vi "chart set up down bars format.vi"(0 "chart":u32, 1 "down_bar_fill":T1, 5 "up_bar_line":T2, 7 "up_bar_fill":T1, 9 "down_bar_line":T2, 11 "error in (no error)":errorcluster) -> (3 "down_bar_fill out":T1, 6 "up_bar_line out":T2, 8 "up_bar_fill out":T1, 10 "down_bar_line out":T2, 15 "error out":errorcluster)   [LabVIEW 2015, in "xlsxwriter.lvlib"]
doc: "void chart_set_up_down_bars_format(lxw_chart chart, lxw_chart_line *up_bar_line, lxw_chart_fill *up_bar_fill, lxw_chart_line *down_bar_line, lxw_chart_fill *down_bar_fill);"
uses:
  xlsxwriter.lvlib
  xlsxwriter.dll
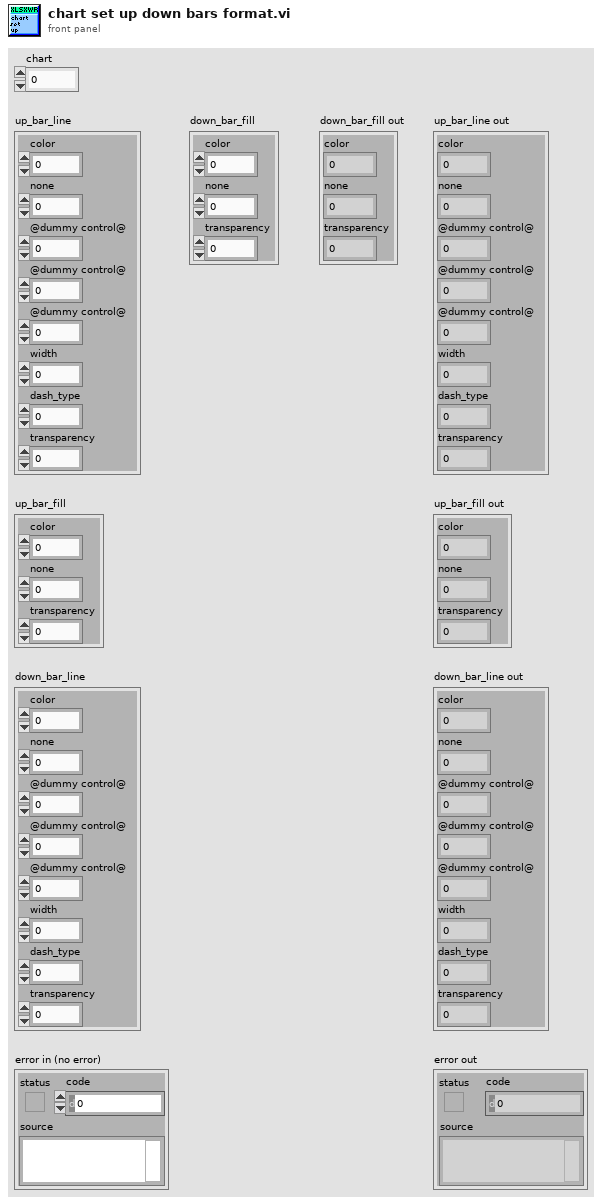
[diagram p1: front panel]
types:
  T1 = cluster{"color":u32, "none":u8, "transparency":u8}
  T2 = cluster{"color":u32, "none":u8, "@dummy control@":i8, "@dummy control@":i8, "@dummy control@":i8, "width":sgl, "dash_type":u8, "transparency":u8}
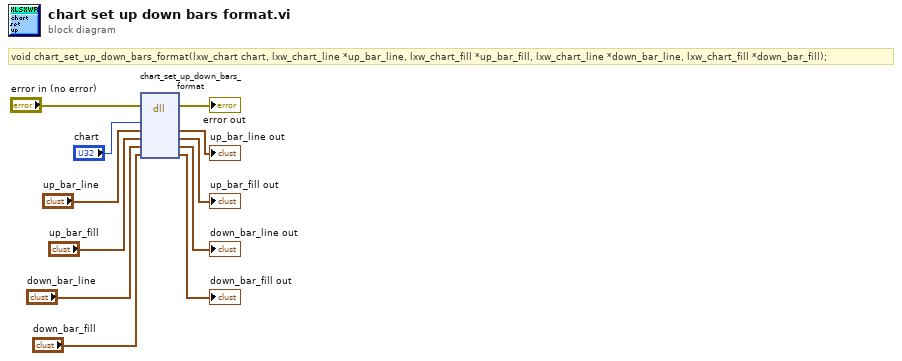
[diagram p0: block diagram]
diagram:
  # "void chart_set_up_down_bars_format(lxw_chart chart, lxw_chart_line *up_bar_line, lxw_chart_fill *up_bar_fill, lxw_chart_line *down_bar_line, lxw_chart_fill *down_bar_fill);"
  n1 = dll-call lib="C:/Users/WDAGUtilityAccount/Desktop/lv_vis_added_cell/xlsxwriter.*" fn="chart_set_up_down_bars_format"(error in="error in (no error)", "chart"="chart", "up_bar_line"="up_bar_line", "up_bar_fill"="up_bar_fill", "down_bar_line"="down_bar_line", "down_bar_fill"="down_bar_fill") -> (error out=→"error out":errorcluster, "up_bar_line"=→"up_bar_line out":T2, "up_bar_fill"=→"up_bar_fill out":T1, "down_bar_line"=→"down_bar_line out":T2, "down_bar_fill"=→"down_bar_fill out":T1)  [unwired: 4 in, 1 out]
